vi "Digital Size.vi"   [LabVIEW 2020]
doc: "Returns the number of samples and signals contained in the digital input. Wire data to the <B>digital waveform in</B> input to determine the polymorphic instance to use or manually select the instance."
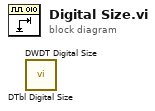
[diagram p0: block diagram]
diagram:
  n1 = call "DTbl Digital Size.vi"() -> ()  [unwired: 8 in, 4 out]
  n2 = call "DWDT Digital Size.vi"() -> ()  [unwired: 8 in, 4 out]
